vi "Adept Device.vi"(0 "Data In":T4, 2 "Display State In":T2, 3 "Container State":T3) -> (6 "Data Out":T4, 7 "Display State Out":T2, 8 "Action":T1)   [LabVIEW 2011, in "LVH-Adept.lvlib" / "Adept Device Ctl.xctl"]
uses:
  Adept Device Ctl.xctl
  Adept Device Data.ctl
  <vilib>/_xctls/Container State.ctl
  Adept Device State.ctl
  <vilib>/_xctls/Action.ctl
  <vilib>/_xctls/XControlSupport.lvlib
panel:
  in  "Device Control":u16(ring)
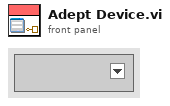
[diagram p1: front panel]
types:
  T1 = typedef "XControlSupport.lvlib/Action.ctl" = cluster{"Data Changed?":bool, "State Changed?":bool, "Action Name":string}
  T2 = typedef "LVH-Adept.lvlib/Adept Device Ctl.xctl/Adept Device State.ctl" = cluster{"Numeric":dbl}
  T3 = typedef "XControlSupport.lvlib/Container State.ctl" = cluster{"Indicator?":bool, "Run Mode?":bool, " Refnum":refnum<vi>}
  T4 = typedef "LVH-Adept.lvlib/Adept Device Ctl.xctl/Adept Device Data.ctl" = u16
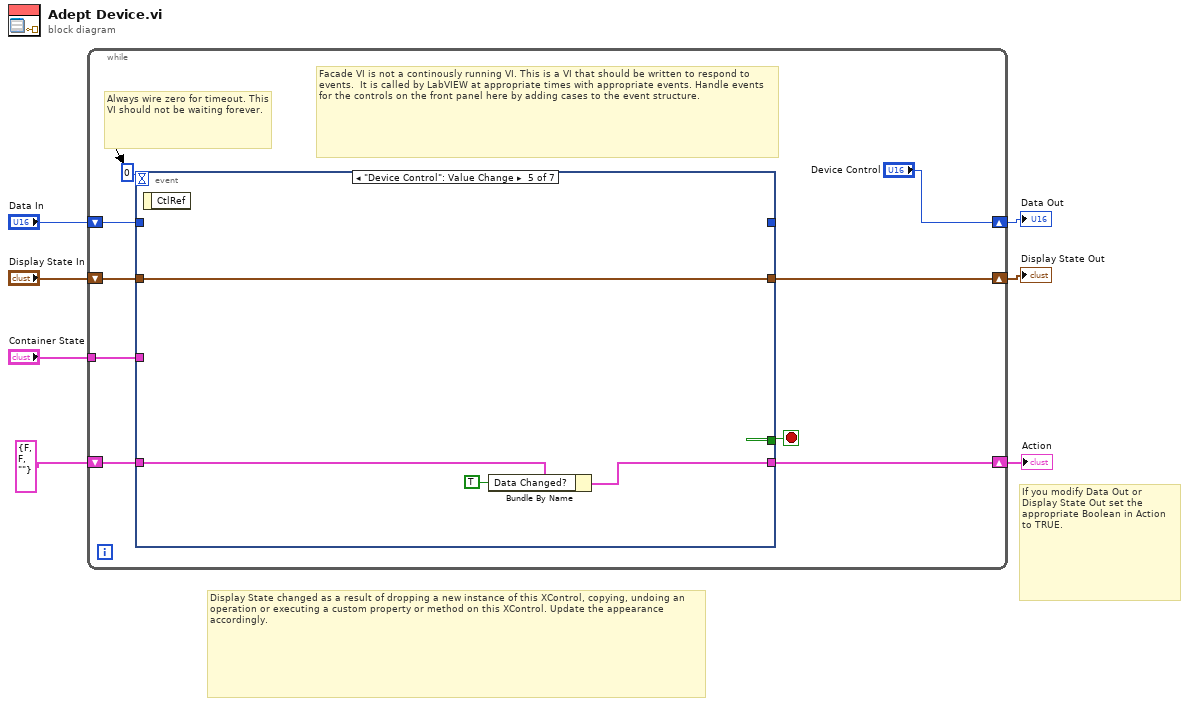
[diagram p0: block diagram]
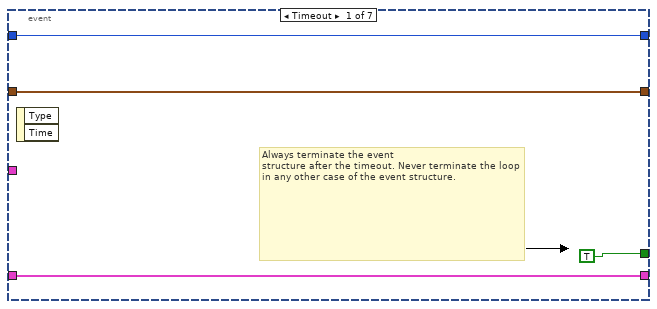
[diagram p2: hidden frame]
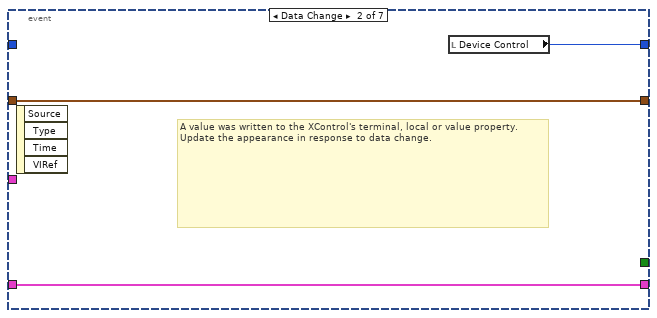
[diagram p3: hidden frame]
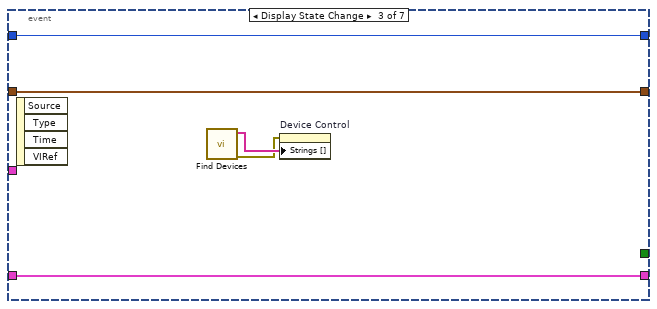
[diagram p4: hidden frame]
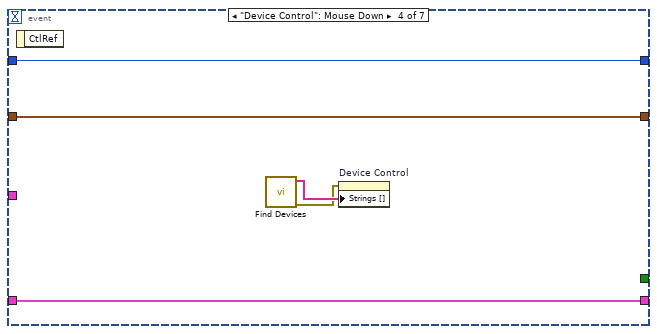
[diagram p5: hidden frame]
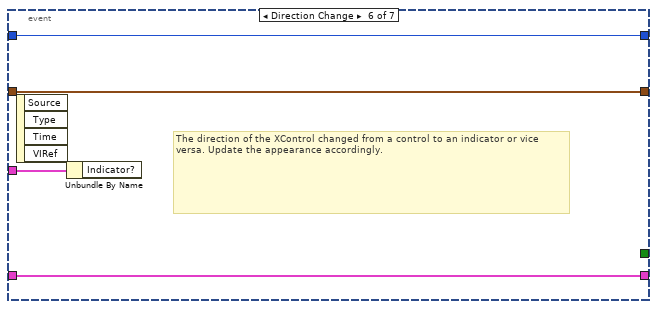
[diagram p6: hidden frame]
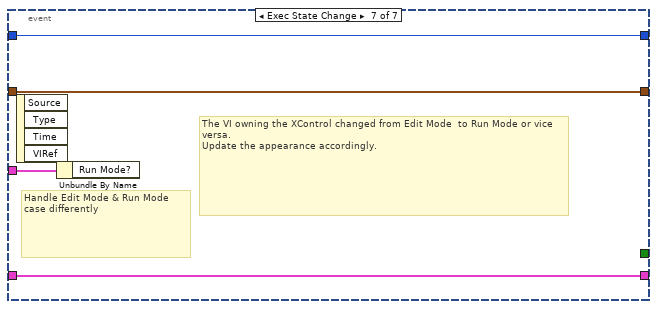
[diagram p7: hidden frame]
diagram:
  # "Display State changed as a result of dropping a new instance of this XControl, copying, undoing an operation or executing a custom property or method on this XControl. Update the appearance accordingly."
  # "If you modify Data Out or\nDisplay State Out set the\nappropriate Boolean in Action\nto TRUE."
  n1 = while {
    shift-right: [w15] -> w4
    shift-left: "Display State In" -> [w16]
    tunnel: "Container State" -> [w12]
    shift-right: ["Device Control"] -> w7
    shift-left: "Data In" -> [w11]
    shift-right: [w9] -> w2
    shift-left: T1 {"Data Changed?"=FALSE, "State Changed?"=FALSE, "Action Name"=""} ("Action") -> [w10]
    stop <- w14 stop-if-true
    # "Facade VI is not a continously running VI. This is a VI that should be written to respond to events.  It is called by LabVIEW at appropriate times with appropriate events. Handle events for the controls on the front panel here by adding cases to the event structure."
    # "Always wire zero for timeout. This\nVI should not be waiting forever."
    n2 = event shown="[4] \"Device Control\": Value Change" {
      selector: _ -> [_ _ _ _ _ _ _]
      dyn-events: _ -> [_ _ _ _ _ _ _]
      timeout: 0 -> [_ _ _ _ _ _ _]
      tunnel: w16 -> [w18 w23 w28 w30 w37 w40 w44]
      tunnel: [w18 w23 w28 w30 w37 w40 w44] -> w15
      tunnel: [TRUE _ _ _ _ _ _] -> w14
      tunnel: w12 -> [_ _ _ _ _ w41 w45]
      tunnel: w11 -> [w17 _ w24 w29 _ w39 w43]
      tunnel: [w17 w21 w24 w29 _ w39 w43] -> _
      tunnel: [w19 w22 w27 w31 w35 w38 w42] -> w9
      tunnel: w10 -> [w19 w22 w27 w31 w36 w38 w42]
      event Timeout {
        # "Always terminate the event\nstructure after the timeout. Never terminate the loop in any other case of the event structure."
        n3 = event-data() -> ()  [unwired: 1 in, 2 out]
      }
      event Data Change {
        # "A value was written to the XControl's terminal, local or value property.\nUpdate the appearance in response to data change."
        n4 = event-data() -> ()  [unwired: 1 in, 4 out]
        n5 = local read "Device Control"() -> (w21:u16)
      }
      event Display State Change {
        n6 = event-data() -> ()  [unwired: 1 in, 4 out]
        n7 = call "Find Devices.vi"() -> ("Error Out"=w25:errorcluster, "Device Names"=w26:string[])  [unwired: 9 in, 1 out]
        n8 = property on="Device Control" class="Ring (strict)"(error in=w25, "Strings []"=w26) -> ()  [unwired: 1 in, 2 out]
      }
      event "Device Control": Mouse Down {
        n9 = event-data() -> ()  [unwired: 1 in, 1 out]
        n10 = call "Find Devices.vi"() -> ("Error Out"=w32:errorcluster, "Device Names"=w33:string[])  [unwired: 9 in, 1 out]
        n11 = property on="Device Control" class="Ring (strict)"(error in=w32, "Strings []"=w33) -> ()  [unwired: 1 in, 2 out]
      }
      event "Device Control": Value Change {
        n12 = event-data() -> ()  [unwired: 1 in, 1 out]
        n13 = Bundle By Name(cluster=w36, "Data Changed?"=TRUE) -> (w35:T1)
      }
      event Direction Change {
        # "The direction of the XControl changed from a control to an indicator or vice versa. Update the appearance accordingly."
        n14 = event-data() -> ()  [unwired: 1 in, 4 out]
        n15 = Unbundle By Name(w41) -> ()  [unwired: 1 out]
      }
      event Exec State Change {
        # "The VI owning the XControl changed from Edit Mode  to Run Mode or vice versa.\nUpdate the appearance accordingly."
        # "Handle Edit Mode & Run Mode\ncase differently"
        n16 = event-data() -> ()  [unwired: 1 in, 4 out]
        n17 = Unbundle By Name(w45) -> ()  [unwired: 1 out]
      }
    }
  }
  "Display State Out" <- w4
  "Data Out" <- w7
  "Action" <- w2
